vi "myRIO__TCP_readAccumParse.vi"(0 "input_strAccum":string, 5 "input_count":i32, 9 "input_handle_TCP":refnum<k5>, 11 "input_error":errorcluster) -> (4 "output_strAccum":string, 6 "output_count":i32, 10 "output_handle_TCP":refnum<k5>, 12 "output_haveCmd":bool, 13 "output_countCmd":i32, 14 "output_strCmd":string, 15 "output_error":errorcluster)   [LabVIEW 2014]
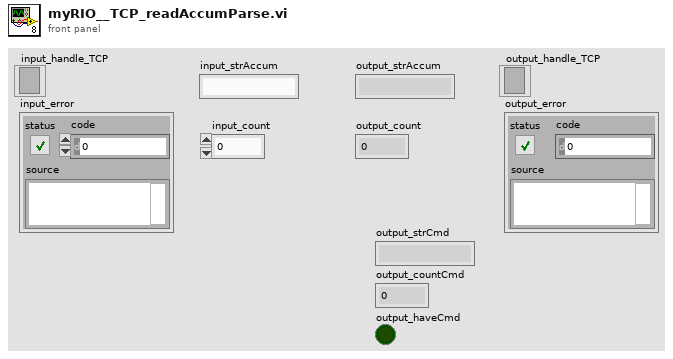
[diagram p1: front panel]
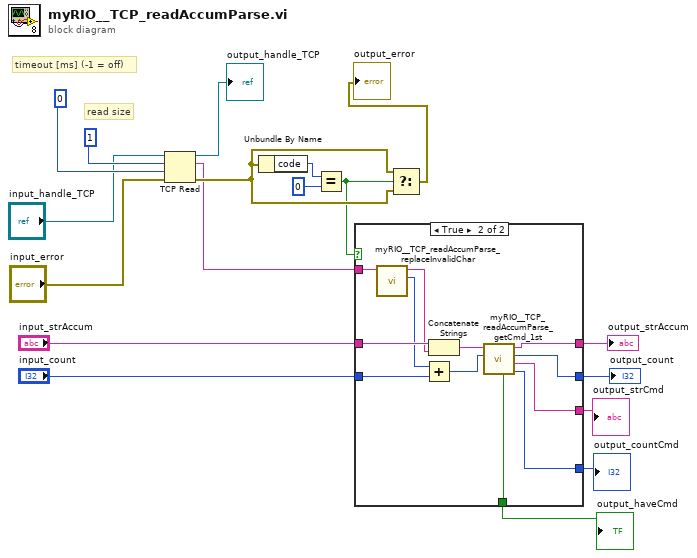
[diagram p0: block diagram]
diagram:
  # "read size"
  # "timeout [ms] (-1 = off)"
  n1 = TCP Read(connection ID="input_handle_TCP", bytes to read=1, error in (no error)="input_error", 9:0 ("timeout ms (25000)")) -> (connection ID out=→"output_handle_TCP":refnum<k5>, data out=w9:string, error out=w11:errorcluster)  [unwired: 1 out]
  n2 = Unbundle By Name(w11) -> ("code"=w13:i32)
  n3 = Equal?(x=w13, y=0) -> (x = y?=w8:bool)
  n4 = case shown="True" w8 {
    tunnel: w9 -> [_ w32]
    tunnel: "input_strAccum" -> [w20 w31]
    tunnel: [w20 w25] -> w6
    tunnel: "input_count" -> [w19 w29]
    tunnel: [w19 w24] -> w4
    tunnel: [_ w23] -> w3
    tunnel: [_ w22] -> w2
    tunnel: [_ w21] -> w1
    frame False {
    }
    frame True {
      n5 = call "myRIO__TCP_readAccumParse_replaceInvalidChar.vi"("input_string"=w32) -> ("output_stringSize"=w28:i32, "output_string"=w30:string)  [unwired: 9 in]
      n6 = Add(x=w28, y=w29) -> (x+y=w26:i32)
      n7 = Concatenate Strings(w31, w30) -> (w27:string)
      n8 = call "myRIO__TCP_readAccumParse_getCmd_1st.vi"("input_count"=w26, "input_strAccum"=w27) -> ("output_countCmd"=w22:i32, "output_strCmd"=w23:string, "output_count"=w24:i32, "output_strAccum"=w25:string, "output_haveCmd"=w21:bool)  [unwired: 5 in]
    }
  }
  "output_strAccum" <- w6
  "output_count" <- w4
  "output_strCmd" <- w3
  "output_countCmd" <- w2
  "output_haveCmd" <- w1
  n9 = Select(t=w11, s=w8, f=w11) -> (s? t:f=→"output_error":errorcluster)
